vi "SinglePoint.vi"(10 "Properties":T1[](array[typedef]), 11 "MeasType":string) -> (3 "Single Point":bool)   [LabVIEW 2017, in "CmsTestPanel.lvlib"]
uses:
  <vilib>/addons/InsightCM/Devices/Shared/Cms/CmsTestPanel/CmsTestPanel.lvlib
  <vilib>/addons/InsightCM/MessageBus/Base/controls/KeyValuePair.ctl
  <vilib>/addons/InsightCM/Utilities/DeviceModelHelpers/DeviceModelHelpers.lvlib
  <vilib>/addons/InsightCM/Utilities/PropertyHelpers/PropertyHelpers.lvlib
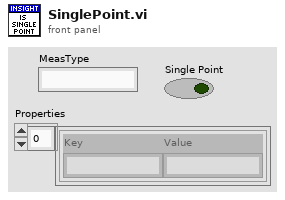
[diagram p1: front panel]
types:
  T1 = typedef "KeyValuePair.ctl" = cluster{"Key":string, "Value":string}
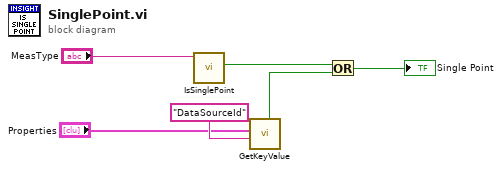
[diagram p0: block diagram]
diagram:
  n1 = call <vilib>:"IsSinglePoint.vi"("MeasType"="MeasType") -> ("is single point"=w4:bool)  [unwired: 10 in]
  n2 = call <vilib>:"GetKeyValue.vi"("key"="DataSourceId" ("name"), "key value pairs"="Properties") -> ("found"=w1:bool)  [unwired: 7 in, 2 out]
  n3 = Or(x=w4, y=w1) -> (x .or. y?=→"Single Point":bool)
